vi "ResampleLUT.vi"(8 "radialsteps":u32, 9 "LUT":sgl[][](array[numeric]), 10 "width":u32, 11 "minRadius":sgl) -> (3 "LUT":dbl[][](array[numeric]))   [LabVIEW 2011]
uses:
  qtrk/QTrkLVBinding/XYZf.ctl
panel:
  out "Radial Profile":sgl[](graph)
  out "Image":sgl[][](graph)
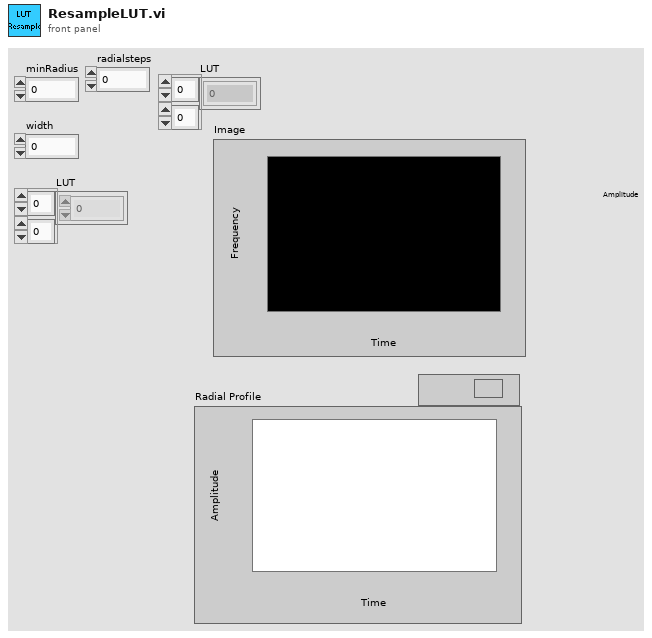
[diagram p1: front panel]
types:
  T1 = typedef "TrackerInstance.ctl" = cluster{"Tracker Pointer":u64, "Image size":cluster{"width":u32, "height":u32}}
  T2 = typedef "XYZf.ctl" = cluster{"X":sgl, "Y":sgl, "Z":sgl}
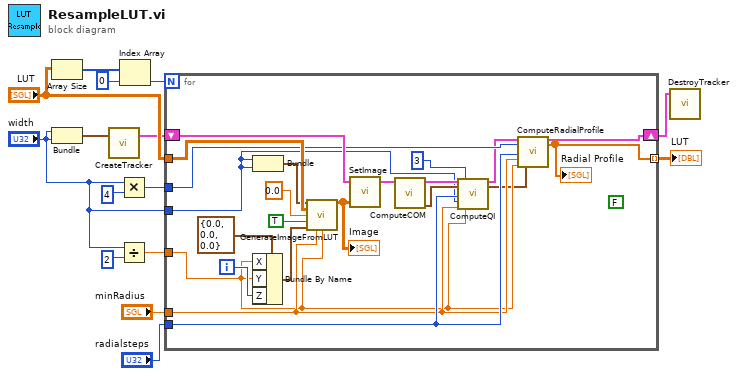
[diagram p0: block diagram]
diagram:
  n1 = Array Size(array="LUT") -> (size(s)=w9:i32[])
  n2 = Bundle("width"="width", "width"="width") -> (w7:cluster{"width":u32, "width":u32})  [unwired: 1 in]
  n3 = call "CreateTracker.vi"("Image size"=w7) -> ("tracker"=w6:T1)  [unwired: 2 in]
  n4 = Multiply(x="width", y=u32 4) -> (x*y=w1:u32)
  n5 = Divide(x="width", y=u32 2) -> (x/y=w12:dbl)
  n6 = Index Array(array=w9, index=0) -> (element=w8:i32)
  n7 = for {
    N: w8 -> [_]
    tunnel: "LUT" -> [w37]
    tunnel: "width" -> [w19]
    tunnel: w12 -> [w17]
    tunnel: "minRadius" -> [w18]
    tunnel: [w26] -> w15 mode=indexing
    shift-right: [w27] -> w5
    shift-left: w6 -> [w29]
    tunnel: "radialsteps" -> [w20]
    tunnel: w1 -> [w25]
    i -> [w35]
    (unwired) FALSE ("Compute Z")
    n8 = Bundle("width"=w19, "width"=w19) -> (w34:cluster{"width":u32, "width":u32})  [unwired: 1 in]
    n9 = Bundle By Name(cluster=T2 {"X"=0.0, "Y"=0.0, "Z"=0.0} ("XYZ"), "X"=w17, "Y"=w17, "Z"=w35) -> (w32:T2)
    n10 = call "GenerateImageFromLUT.vi"("Image Size"=w34, "ZLUT"=w37, "Pixel max value"=sgl 0.0, "Use spline interpolation?"=TRUE, "XYZ"=w32, "ZLUT MinRadius"=w18, "ZLUT MaxRadius"=w17) -> ("Result image"=w30:sgl[][])  [unwired: 8 in]
    "Image" <- w30
    n11 = call "SetImage.vi"("tracker"=w29, "Image (float)"=w30) -> ("tracker"=w28:T1)  [unwired: 6 in, 1 out]
    n12 = call "ComputeCOM.vi"("tracker"=w28) -> ("position"=w24:cluster{"X":sgl, "Y":sgl}, "tracker"=w23:T1)  [unwired: 5 in]
    n13 = call "ComputeQI.vi"("tracker"=w23, "initial position"=w24, "radialSteps"=w20, "angularStepsPerQuadrant"=w19, "minRadius"=w18, "iterations"=3, "maxRadius"=w17) -> ("tracker"=w22:T1, "position"=w16:cluster{"X":sgl, "Y":sgl})  [unwired: 10 in, 1 out]
    n14 = call "ComputeRadialProfile.vi"("tracker"=w22, "angularSteps"=w25, "radialsteps"=w20, "minradius"=w18, "maxradius"=w17, "center"=w16) -> ("tracker"=w27:T1, "output"=w26:sgl[])  [unwired: 11 in, 1 out]
    "Radial Profile" <- w26
  }
  "LUT" <- w15
  n15 = call "DestroyTracker.vi"("tracker instance"=w5) -> ()  [unwired: 5 in]
